vi "ndipolaris Read Transformations.vi"(6 "Track Outside Measurement Volume? (F:No)":bool, 8 "error in (no error)":errorcluster, 9 "Track Stray Markers? (F:No)":bool, 10 "Get Extended Tool Info? (F:No)":bool, 11 "VISA resource name":refnum<visa-resource-name>) -> (0 "error out":errorcluster, 1 "Extended Information":T1(array[cluster]), 2 "Transformations":T2(array[cluster]), 3 "VISA resource out":refnum<visa-resource-name>)   [LabVIEW 2013]
doc: "This VI will send a command to the Polaris instrument requesting a transform. The transform is returned in Tool Info Array, where each index of Tool Info Array is a transformation for a different tool (the tool is referenced by Port Handle). The instrument must be in the Tracking state to acquire transformations."
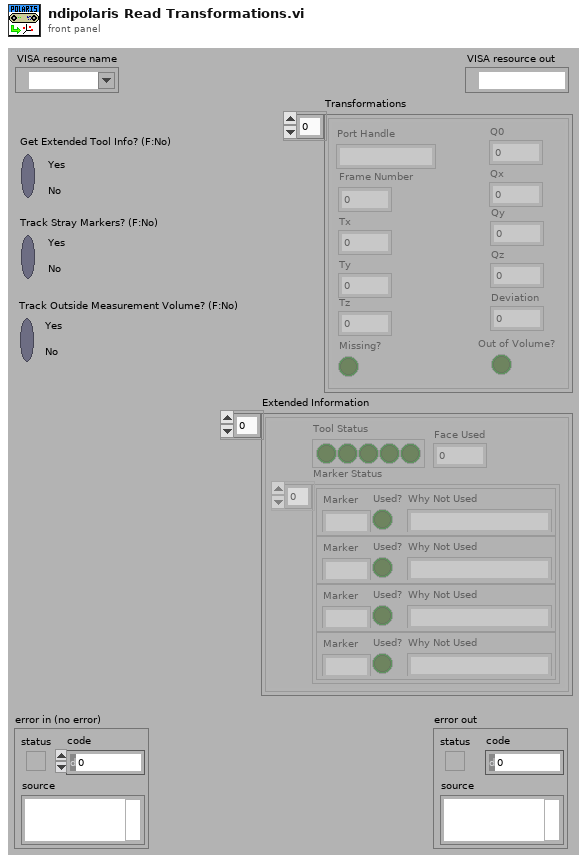
[diagram p1: front panel]
types:
  T1 = cluster{"Tool Status":bool[], "Face Used":i32, "Marker Status":cluster{"Marker":string, "Used?":bool, "Why Not Used":string}[]}[]
  T2 = cluster{"Port Handle":string, "Frame Number":u32, "Tx":dbl, "Ty":dbl, "Tz":dbl, "Q0":dbl, "Qx":dbl, "Qy":dbl, "Qz":dbl, "Deviation":dbl, "Missing?":bool, "Out of Volume?":bool}[]
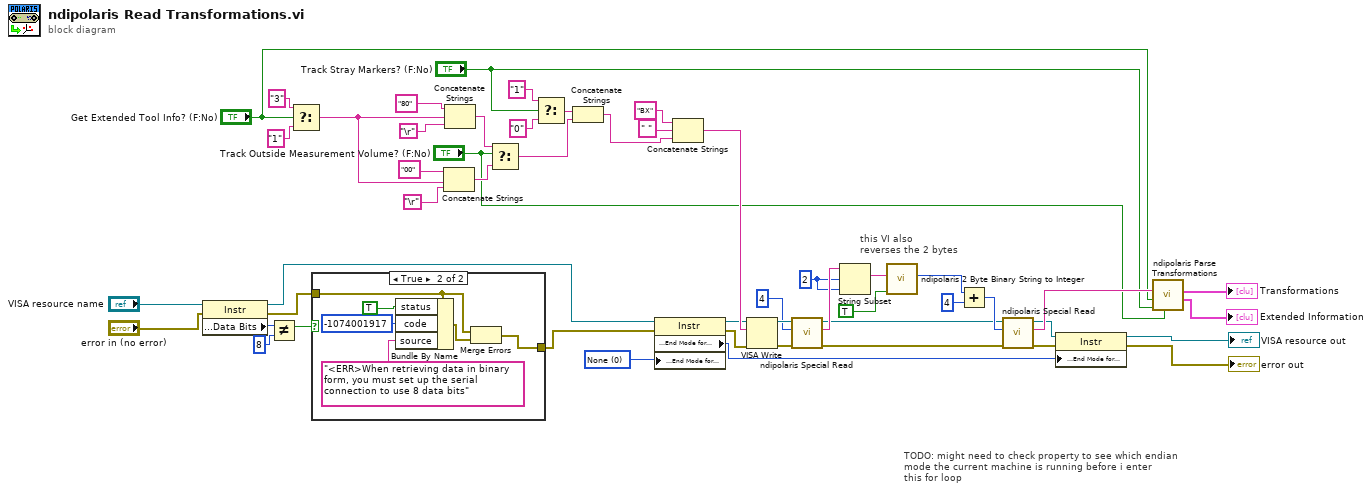
[diagram p0: block diagram]
diagram:
  w28 = 2 ("offset (0)")
  w31 = u16 0 items=["None", "LastBit", "TermChar"] ("Serial Settings:Serial End Mode for Reads")
  # "this VI also\nreverses the 2 bytes"
  # "TODO: might need to check property to see which endian\nmode the current machine is running before i enter\nthis for loop"
  n1 = property on="Property Node" class="Instr"(reference="VISA resource name", error in="error in (no error)") -> (reference out=w40:refnum<visa-resource-name>, error out=w42:errorcluster, "Serial Settings:Data Bits"=w44:u16)
  n2 = Not Equal?(x=w44, y=u16 8) -> (x != y?=w41:bool)
  n3 = Select(t="3", s="Get Extended Tool Info? (F:No)", f="1") -> (s? t:f=w5:string)
  n4 = case shown="True" w41 {
    tunnel: w42 -> [w52 w53]
    tunnel: [w52 w57] -> w10
    frame False {
    }
    frame True {
      n5 = Bundle By Name(cluster=w53, "status"=TRUE, "code"=-1074001917, "source"="<ERR>When retrieving data in binary form, you must set up the serial connection to use 8 data bits") -> (w58:errorcluster)
      n6 = Merge Errors(w53, w58) -> (w57:errorcluster)
    }
  }
  n7 = Concatenate Strings("00" ("string"), w5, "\r" ("Carriage Return Constant")) -> (w17:string)
  n8 = Concatenate Strings("80", w5, "\r" ("Carriage Return Constant")) -> (w19:string)
  n9 = Select(t=w19, s="Track Outside Measurement Volume? (F:No)", f=w17) -> (s? t:f=w16:string)
  n10 = Select(t="1", s="Track Stray Markers? (F:No)", f="0") -> (s? t:f=w15:string)
  n11 = Concatenate Strings(w15, w16) -> (w11:string)
  n12 = property on="Property Node" class="Instr"(reference=w40, error in=w10, "Serial Settings:End Mode for Reads"=w31) -> (reference out=w39:refnum<visa-resource-name>, error out=w38:errorcluster, "Serial Settings:End Mode for Reads"=w30:u16)
  n13 = Concatenate Strings("BX" ("string"), " " ("string"), w11) -> (w45:string)
  n14 = VISA Write(VISA resource name=w39, write buffer=w45, error in (no error)=w38) -> (VISA resource name out=w37:refnum<visa-resource-name>, error out=w36:errorcluster)  [unwired: 1 out]
  n15 = call <instrlib>:"ndipolaris Special Read.vi"("error in (no error)"=w36, "Bytes to Read (100)"=u32 4 ("byte count"), "VISA resource name"=w37) -> ("error out"=w23:errorcluster, "read buffer"=w29:string, "VISA resource out"=w24:refnum<visa-resource-name>)  [unwired: 6 in]
  n16 = String Subset(string=w29, offset (0)=w28, length (rest)=w28) -> (substring=w27:string)
  n17 = call <instrlib>:"ndipolaris 2 Byte Binary String to Integer.vi"("Perform Byte Switch? (T:Yes)"=TRUE ("Perform Byte Switch? (T)"), "String to Convert"=w27) -> ("Converted Integer"=w26:u16)  [unwired: 9 in]
  n18 = Add(x=w26, y=u32 4) -> (x+y=w25:u32)
  n19 = call <instrlib>:"ndipolaris Special Read.vi"("error in (no error)"=w23, "Bytes to Read (100)"=w25, "VISA resource name"=w24) -> ("error out"=w32:errorcluster, "read buffer"=w46:string, "VISA resource out"=w33:refnum<visa-resource-name>)  [unwired: 6 in]
  n20 = property on="Property Node" class="Instr"(reference=w33, error in=w32, "Serial Settings:End Mode for Reads"=w30) -> (reference out=→"VISA resource out":refnum<visa-resource-name>, error out=→"error out":errorcluster)
  n21 = call <instrlib>:"ndipolaris Parse Transformations.vi"("Track Outside Measurement Volume? (F:No)"="Track Outside Measurement Volume? (F:No)", "Track Stray Markers? (F:No)"="Track Stray Markers? (F:No)", "Get Extended Tool Info? (F:No)"="Get Extended Tool Info? (F:No)", "Transformation String"=w46) -> ("Extended Information"=→"Extended Information":T1, "Transformations"=→"Transformations":T2)  [unwired: 6 in]
